vi "Restarts Monitor (RT).vi"() -> ()   [LabVIEW 2013]
uses:
  <vilib>/FPGAPlugInAG/sbRIO-9626/niLvFpga_Open_sbRIO-9626.vi
  <vilib>/rvi/interface/common/dynamic/niFpgaDynamicAddResources.vi
  <vilib>/FPGAPlugInAG/Dynamic/niLvFpga_Reset_Dynamic.vi
  <vilib>/FPGAPlugInAG/Dynamic/niLvFpga_Run_Dynamic.vi
  <vilib>/rvi/interface/common/niFpgaWaitOnOcc.vi
  <vilib>/Utility/error.llb/Error Cluster From Error Code.vi
  <vilib>/rvi/errors/niLvFpgaAdjustHostInterfaceError.vi
  <vilib>/rvi/interface/nirviOpenFPGA/nirviOpenFPGA.xnode
  FPGA Bitfiles/TIsbRIO_FPGATarget_RestartsMonitor(_OLXcOrNoyY8.lvbitx
  FPGA/Restarts Monitor (FPGA).vi
  <vilib>/rvi/interface/nirviMethod/nirviMethod.xnode
  <vilib>/rvi/interface/nirviReadWriteControl/nirviReadWriteControl.xnode
  <vilib>/NI_Real-Time Target Support.lvlib
  NiFpgaLv.dll
  <vilib>/rvi/interface/Simulation/niFpgaSimulationCallBeginRW.vi
panel:
  out "Restarts":i32[](array[numeric])
  in  "Reset":bool
  out "CPU (%)":dbl
  out "Commanded Starts":u32
  out "error out":errorcluster
  out "Actual Starts":u32[](array[numeric])
  in  "Loop Timer (uSec)":u32=400
  in  "Consec Samples":i32=125
  in  "Threshold (A)":sgl=1.0
  # "Pump 1"
  # "Pump 2"
  # "Pump 3"
  # "Pump 4"
  # "Pump 5"
  # "Pump 6"
  # "Pump 7"
  # "Pump 8"
  # "Pump 9"
  # "Pump 10"
  # "Pump 11"
  # "Pump 12"
  # "[Actual Starts] - [Commanded Starts] = [Restarts]"
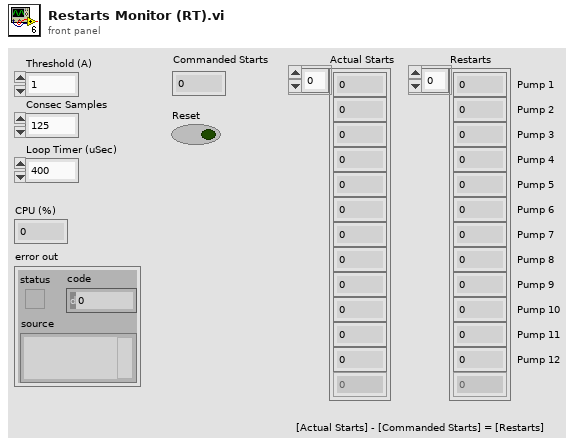
[diagram p1: front panel]
types:
  T1 = typedef "CANFrameControl.ctl" = cluster{"identifier":u32, "extended?":bool, "type":enum8{"CAN Data", "CAN Remote"}, "payload":u8[]}
  T2 = typedef "NI_Real-Time Target Support.lvlib/RT CPU Load.ctl" = cluster{"Total (%)":dbl, "Time Critical (%)":dbl, "Timed Structures (%)":dbl, "High (%)":dbl, "Above Normal (%)":dbl, "Normal (%)":dbl, "Background (%)":dbl, "Idle (%)":dbl, "ISR (%)":dbl}
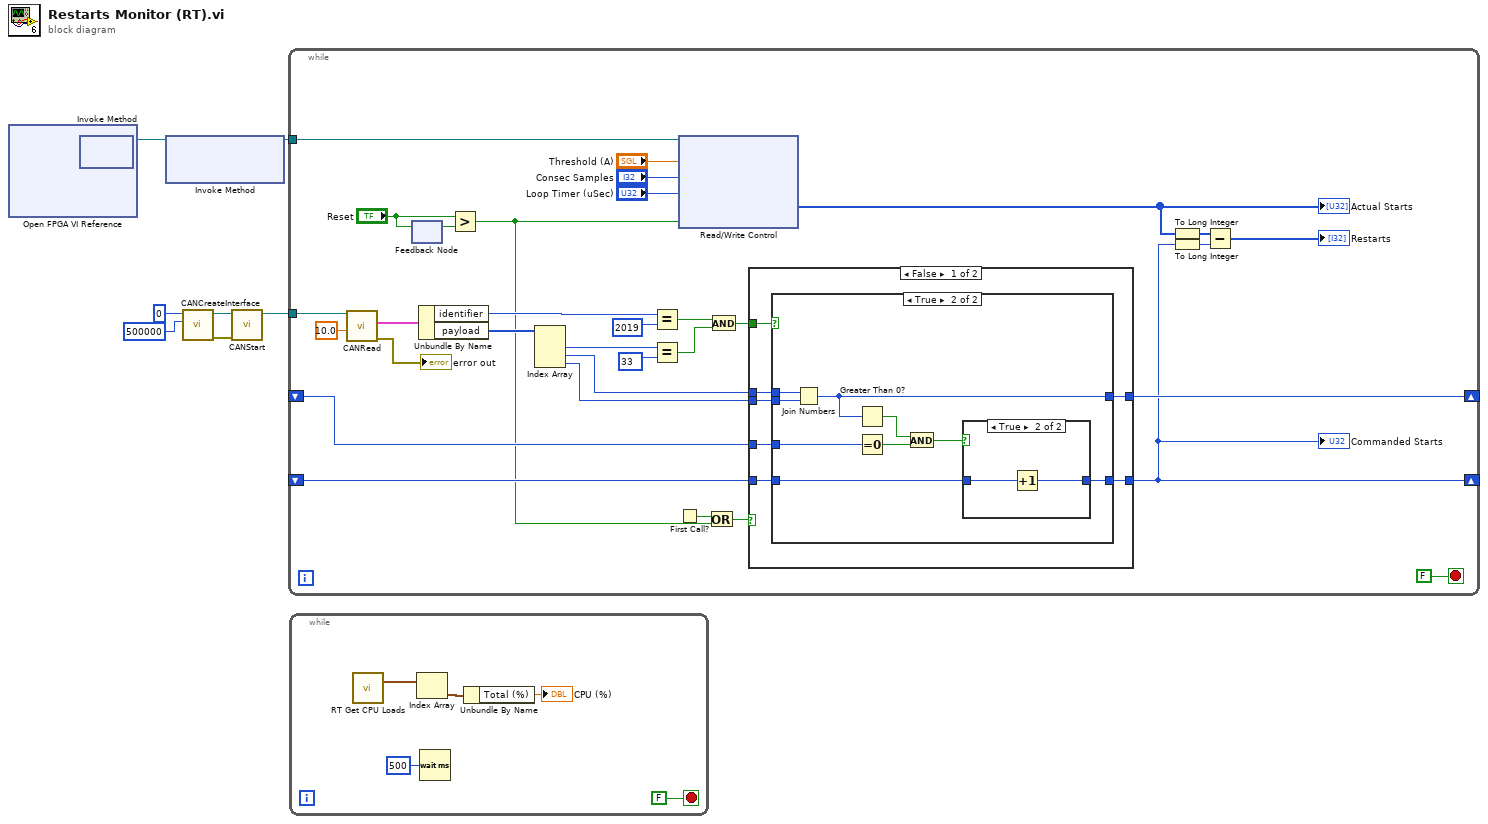
[diagram p0: block diagram]
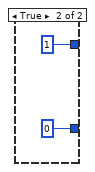
[diagram p4: hidden frame]
diagram:
  n1 = xnode "Open FPGA VI Reference"() -> ("FPGA VI Reference Out"=w3:refnum<k20>)  [unwired: 2 in, 1 out]
  n2 = xnode "Invoke Method"("FPGA VI Reference In"=w3) -> ("FPGA VI Reference Out"=w2:refnum<k20>)  [unwired: 1 in, 1 out]
  n3 = xnode "Invoke Method"("FPGA VI Reference In"=w2) -> ("FPGA VI Reference Out"=w1:refnum<k20>)  [unwired: 2 in, 1 out]
  n4 = call <vilib>:"CANCreateInterface.vi"("baud rate"=u32 500000, "interface index"=u32 0) -> ("error out"=w8:errorcluster, "interface object out"=w7:refnum<k20>)  [unwired: 8 in]
  n5 = call <vilib>:"CANStart.vi"("error in (no error)"=w8, "interface object in"=w7) -> ("interface object out"=w4:refnum<k20>)  [unwired: 8 in, 1 out]
  n6 = while {
    tunnel: w1 -> [w40]
    tunnel: w4 -> [w35]
    shift-right: [w21] -> _
    shift-left: _ -> [w20]
    shift-right: [w12] -> _
    shift-left: _ -> [w19]
    stop <- FALSE stop-if-true
    n7 = call <vilib>:"CANRead.vi"("timeout"=10.0, "interface object in"=w35) -> ("error out"=→"error out":errorcluster, "CAN frame"=w33:T1)  [unwired: 6 in, 2 out]
    n8 = feedback-in #1("Reset") -> ()
    n9 = feedback #1() -> (w17:bool)  [unwired: 1 in]
    n10 = Unbundle By Name(w33) -> ("identifier"=w31:u32, "payload"=w32:u8[])
    n11 = Greater?(x="Reset", y=w17) -> (0:w15:bool)
    n12 = Index Array(array=w32) -> (element #1=w29:u8, element #2=w24:u8, element #3=w23:u8)  [unwired: 3 in]
    n13 = Equal?(x=w31, y=u32 2019) -> (x = y?=w27:bool)
    n14 = Equal?(x=w29, y=u8 33 ("y 2")) -> (x = y?=w26:bool)
    n15 = First Call?() -> (First Call?: T/F=w16:bool)
    n16 = xnode "Read/Write Control"("FPGA VI Reference In"=w40, "Threshold (A)"="Threshold (A)", "Consec Samples"="Consec Samples", "Loop Timer (uSec)"="Loop Timer (uSec)", "Reset"=w15) -> ("Actual Pump Starts"=w13:u32[])  [unwired: 1 in, 2 out]
    "Actual Starts" <- w13
    n17 = Or(x=w16, y=w15) -> (x .or. y?=w14:bool)
    n18 = And(x=w27, y=w26) -> (x .and. y?=w22:bool)
    n19 = case shown="False" w14 {
      tunnel: w24 -> [w47 _]
      tunnel: w23 -> [w46 _]
      tunnel: w22 -> [w45 _]
      tunnel: [w44 u16 1] -> w21
      tunnel: w20 -> [w43 _]
      tunnel: w19 -> [w42 _]
      tunnel: [w41 u32 0] -> w12
      frame False {
        n20 = case shown="True" w45 {
          tunnel: w47 -> [_ w58]
          tunnel: w46 -> [_ w57]
          tunnel: [w49 w55] -> w44
          tunnel: w43 -> [w49 w56]
          tunnel: w42 -> [w48 w51]
          tunnel: [w48 w50] -> w41
          frame False {
          }
          frame True {
            n21 = Join Numbers(hi=w58, lo=w57) -> ((hi.lo)=w55:u16)
            n22 = Greater Than 0?(x=w55) -> (x > 0?=w54:bool)
            n23 = Equal To 0?(x=w56) -> (x = 0?=w53:bool)
            n24 = And(x=w54, y=w53) -> (x .and. y?=w52:bool)
            n25 = case shown="True" w52 {
              tunnel: w51 -> [w59 w61]
              tunnel: [w59 w60] -> w50
              frame False {
              }
              frame True {
                n26 = Increment(x=w61) -> (x+1=w60:u32)
              }
            }
          }
        }
      }
      frame True {
      }
    }
    "Commanded Starts" <- w12
    n27 = To Long Integer(number=w13) -> (32bit integer=w11:i32[])
    n28 = To Long Integer(number=w12) -> (32bit integer=w10:i32)
    n29 = Subtract(x=w11, y=w10) -> (x-y=→"Restarts":i32[])
  }
  n30 = while {
    stop <- FALSE stop-if-true
    n31 = call <vilib>:"RT Get CPU Loads.vi"() -> ("CPU loads"=w67:T2[])  [unwired: 10 in, 1 out]
    n32 = Index Array(array=w67) -> (element=w66:T2)  [unwired: 1 in]
    n33 = Wait (ms)(milliseconds to wait=u32 500) -> ()  [unwired: 1 out]
    n34 = Unbundle By Name(w66) -> ("Total (%)"=→"CPU (%)":dbl)
  }
